vi "Configure Trigger (State).vi"(0 "VISA resource name":refnum<visa-resource-name>, 1 "Trigger Condition (0:False)":u16(ring) items=["False", "True"], 2 "Trigger Event (0:A Event)":u16(ring) items=["A Event", "B Event"], 5 "Channel1 Input":T4={"Channel1 Logical Input (0:High)"=0, "Channel1 Threshold (1.0v)"=1.0} {"Channel1 Logical Input (0:High)" items=["High", "Low", "X"]}, 7 "Channel2 Input":T3={"Channel2 Logical Input (0:High) "=0, "Channel2 Threshold (1.0v) "=1.0} {"Channel2 Logical Input (0:High)" items=["High", "Low", "X"]}, 9 "Pattern Type (0:AND)":u16(ring) items=["AND", "NAND", "OR", "NOR"], 11 "error in (no error)":errorcluster, 12 "Channel3 Input":T2={"Channel3 Logical Input (0:High)"=0, "Channel3 Threshold (1.0v)"=1.0} {"Channel3 Logical Input (0:High)" items=["High", "Low", "X"]}, 13 "Channel4 Input":T1={"Channel4 Logical Input (0:Positive)"=0, "Channel4 Threshold (1.0v)"=1.0} {"Channel4 Logical Input (0:Positive)" items=["Positive", "Negative"]}) -> (4 "VISA resource name out":refnum<visa-resource-name>, 15 "error out":errorcluster)   [LabVIEW 2012, in "Tektronix 7000 Series.lvlib"]
doc: "Configures state trigger settings for an oscilloscope. For a 4-channel oscilloscope, a state occurs when the specified conditions of Channels 1, 2, and 3 are met after the Channel 4 clock condition is met. For a 2-channel oscilloscope, a state occurs when the specified conditions of channel 1 are met after the Channel 2 clock condition is met.\n\nTDS5000,TDS5000B,TDS6000,CSA7000 and TDS7000 series oscilloscopes don't support B State Trigger."
uses:
  Tektronix 7000 Series.lvlib
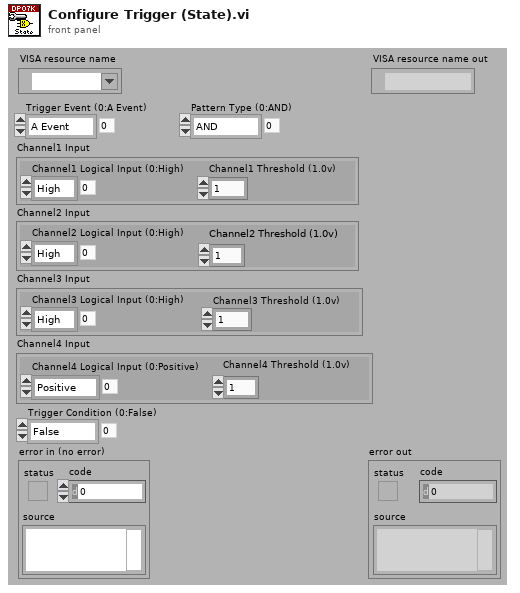
[diagram p1: front panel]
types:
  T1 = cluster{"Channel4 Logical Input (0:Positive)":u16, "Channel4 Threshold (1.0v)":dbl}
  T2 = cluster{"Channel3 Logical Input (0:High)":u16, "Channel3 Threshold (1.0v)":dbl}
  T3 = cluster{"Channel2 Logical Input (0:High) ":u16, "Channel2 Threshold (1.0v) ":dbl}
  T4 = cluster{"Channel1 Logical Input (0:High)":u16, "Channel1 Threshold (1.0v)":dbl}
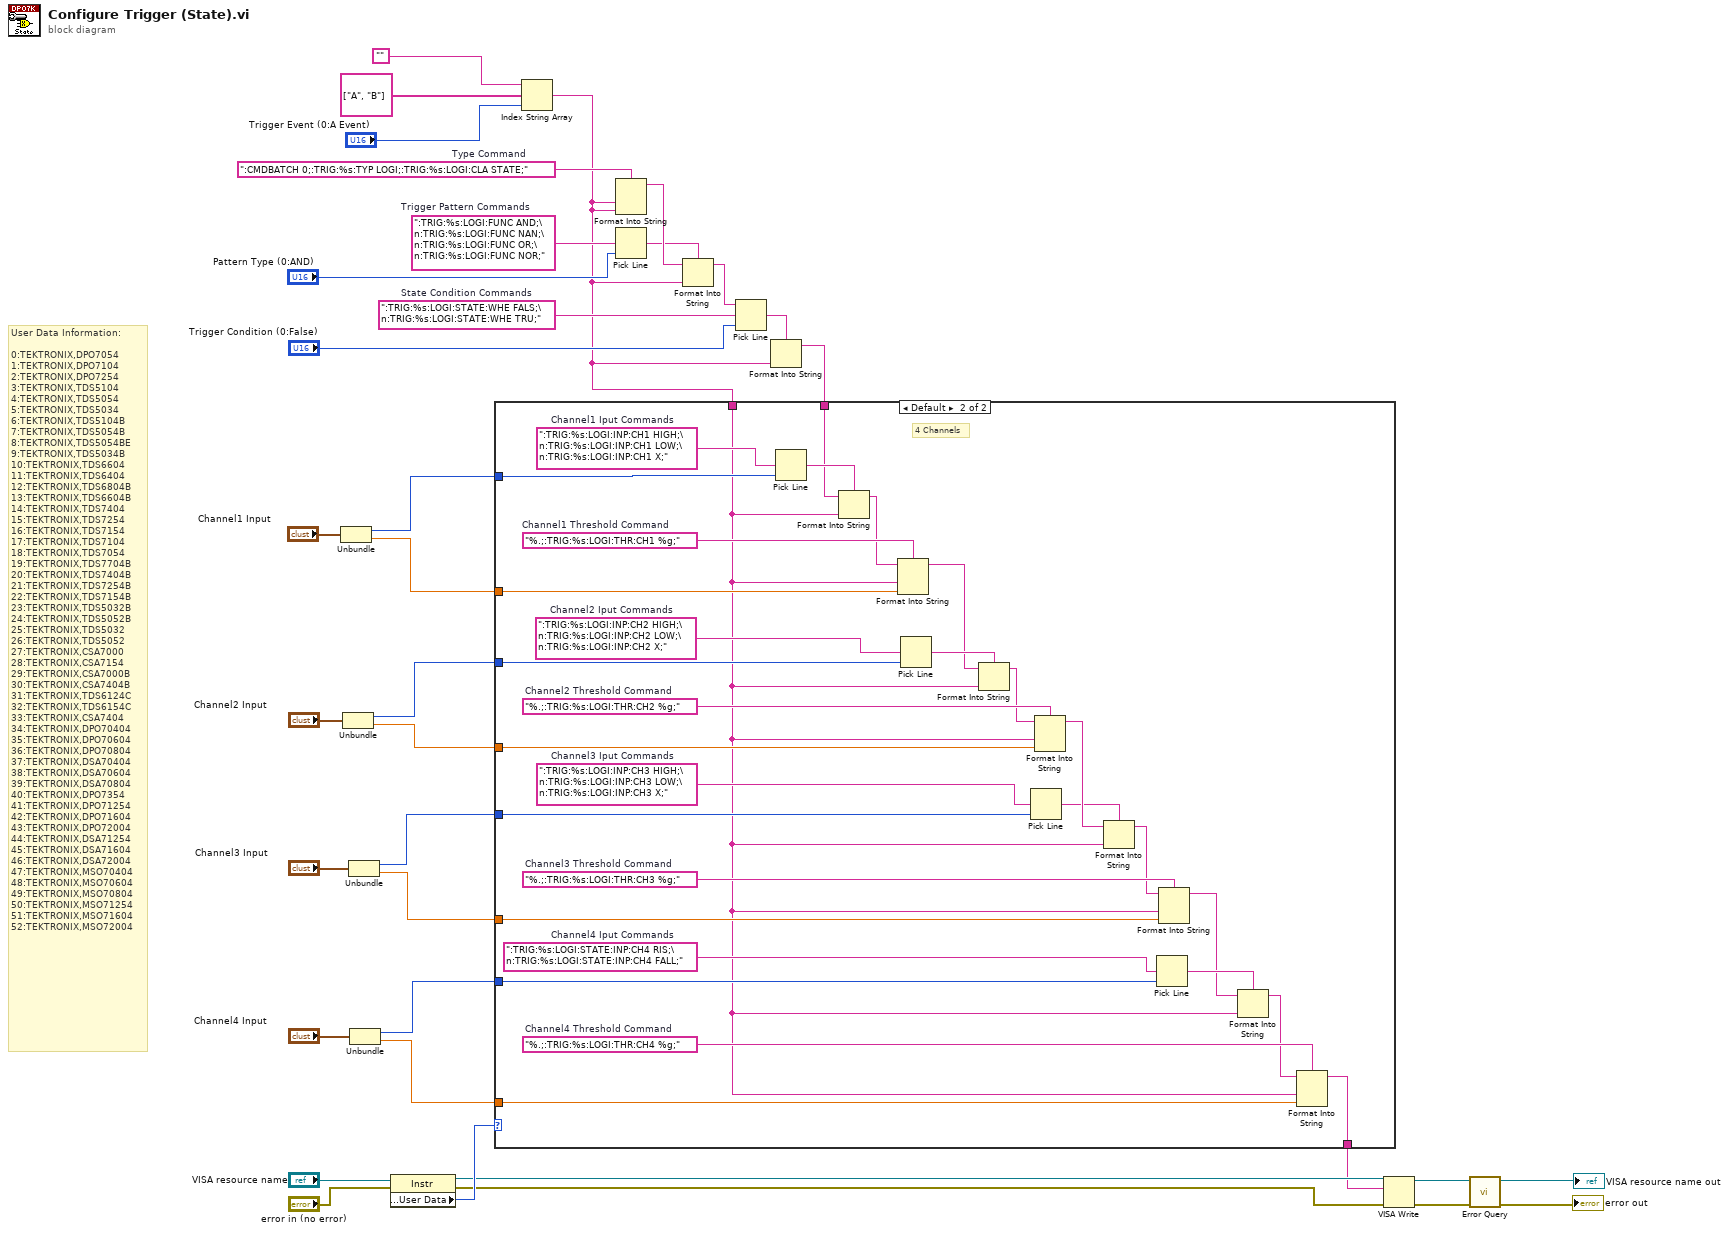
[diagram p0: block diagram]
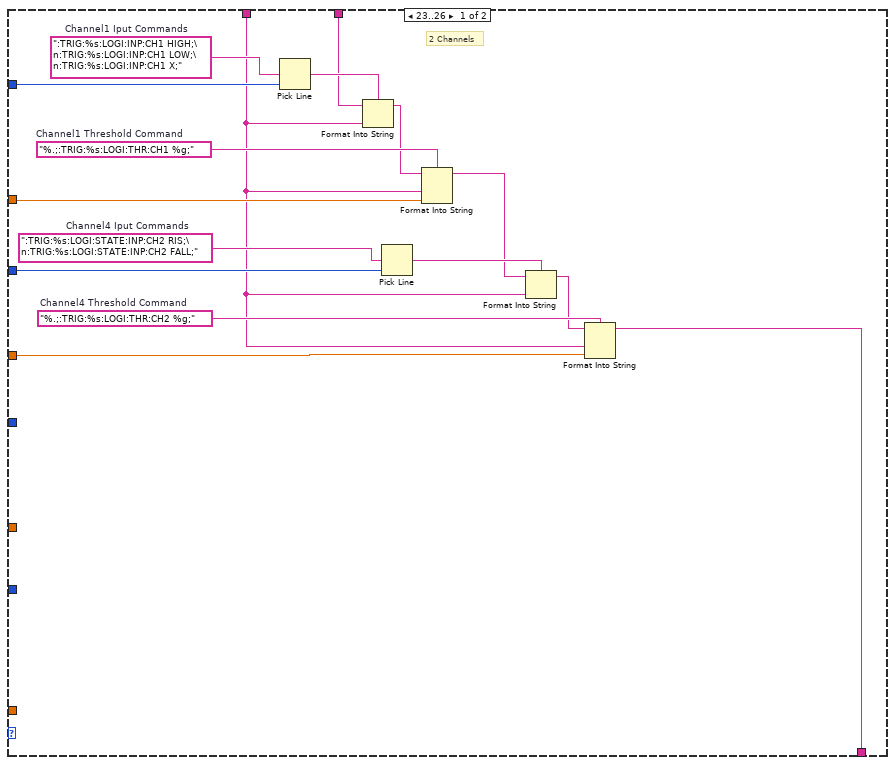
[diagram p2: hidden frame]
diagram:
  w18 = ":TRIG:%s:LOGI:STATE:WHE FALS;\n:TRIG:%s:LOGI:STATE:WHE TRU;"  # State Condition Commands
  w19 = ":TRIG:%s:LOGI:FUNC AND;\n:TRIG:%s:LOGI:FUNC NAN;\n:TRIG:%s:LOGI:FUNC OR;\n:TRIG:%s:LOGI:FUNC NOR;"  # Trigger Pattern Commands
  w17 = ":CMDBATCH 0;:TRIG:%s:TYP LOGI;:TRIG:%s:LOGI:CLA STATE;"  # Type Command
  # "User Data Information:\n\n0:TEKTRONIX,DPO7054\n1:TEKTRONIX,DPO7104\n2:TEKTRONIX,DPO7254\n3:TEKTRONIX,TDS5104\n4:TEKTRONIX,TDS5054\n5:TEKTRONIX,TDS5034\n6:TEKTRONIX,TDS5104B\n7:TEKTRONIX,TDS5054B\n8:TEKTRONIX,TDS5054BE\n9:TEKTRONIX,TDS5034B\n10:TEKTRONIX,TDS6604\n11:TEKTRONIX,TDS6404\n12:TEKTRONIX,TDS6804B\n13:TEKTRONIX,TDS6604B\n14:TEKTRONIX,TDS7404\n15:TEKTRONIX,TDS7254\n16:TEKTRONIX,TDS7154\n17:TEKTRONIX,TDS7104\n18:TEKTRONIX,TDS7054\n19:TEKTRONIX,TDS7704B\n20:TEKTRONIX,TDS7404B\n21:TEKTRONIX,TDS7254B\n22:TEKTRONIX,TDS7154B\n23:TEKTRONIX,TDS5032B\n24:TEKTRONIX,TDS5052B\n25:TEKTRONIX,TDS5032\n26:TEKTRONIX,TDS5052\n27:TEKTRONIX,CSA7000\n28:TEKTRONIX,CSA7154\n29:TEKTRONIX,CSA7000B\n30:TEKTRONIX,CSA7404B\n31:TEKTRONIX,TDS6124C\n32:TEKTRONIX,TDS6154C\n33:TEKTRONIX,CSA7404\n34:TEKTRONIX,DPO70404\n35:TEKTRONIX,DPO70604\n36:TEKTRONIX,DPO70804\n37:TEKTRONIX,DSA70404\n38:TEKTRONIX,DSA70604\n39:TEKTRONIX,DSA70804\n40:TEKTRONIX,DPO7354\n41:TEKTRONIX,DPO71254\n42:TEKTRONIX,DPO71604\n43:TEKTRONIX,DPO72004\n44:TEKTRONIX,DSA71254\n45:TEKTRONIX,DSA71604\n46:TEKTRONIX,DSA72004\n47:TEKTRONIX,MSO70404\n48:TEKTRONIX,MSO70604\n49:TEKTRONIX,MSO70804\n50:TEKTRONIX,MSO71254\n51:TEKTRONIX,MSO71604\n52:TEKTRONIX,MSO72004"
  n1 = Unbundle("Channel1 Input") -> ("Channel1 Logical Input (0:High)"=w34:u16, "Channel1 Threshold (1.0v)"=w14:dbl)
  n2 = Unbundle("Channel2 Input") -> ("Channel2 Logical Input (0:High)"=w32:u16, "Channel2 Threshold (1.0v)"=w13:dbl)
  n3 = Unbundle("Channel3 Input") -> ("Channel3 Logical Input (0:High)"=w30:u16, "Channel3 Threshold (1.0v)"=w12:dbl)
  n4 = Unbundle("Channel4 Input") -> ("Channel4 Logical Input (0:Positive)"=w28:u16, "Channel4 Threshold (1.0v)"=w11:dbl)
  n5 = property class="Instr"(reference="VISA resource name", error in="error in (no error)") -> (reference out=w4:refnum<visa-resource-name>, error out=w3:errorcluster, "General Settings:User Data"=w5:u32)
  n6 = Index String Array(1:"Trigger Event (0:A Event)", 2:string[] ["A", "B"], 3:"" ("Empty String Constant")) -> (0:w8:string)
  n7 = Format Into String(format string=w17, w8, w8) -> (resulting string=w16:string)  [unwired: 2 in, 1 out]
  n8 = Pick Line(multi-line string=w19, line index="Pattern Type (0:AND)") -> (output string=w15:string)  [unwired: 1 in]
  n9 = Format Into String(format string=w15, initial string=w16, w8) -> (resulting string=w9:string)  [unwired: 1 in, 1 out]
  n10 = Pick Line(string ("")=w9, multi-line string=w18, line index="Trigger Condition (0:False)") -> (output string=w10:string)
  n11 = Format Into String(format string=w10, w8) -> (resulting string=w1:string)  [unwired: 2 in, 1 out]
  n12 = case shown="Default" w5 {
    tunnel: w34 -> [w48 w82]
    tunnel: w32 -> [w41 w81]
    tunnel: w30 -> [_ w80]
    tunnel: w28 -> [_ w79]
    tunnel: w14 -> [w47 w68]
    tunnel: w13 -> [w42 w64]
    tunnel: w12 -> [_ w60]
    tunnel: w11 -> [_ w56]
    tunnel: w8 -> [w40 w55]
    tunnel: [w38 w54] -> w2
    tunnel: w1 -> [w37 w53]
    frame 23..26 {
      w46 = "%.;:TRIG:%s:LOGI:THR:CH2 %g;"  # Channel4 Threshold Command
      w45 = ":TRIG:%s:LOGI:STATE:INP:CH2 RIS;\n:TRIG:%s:LOGI:STATE:INP:CH2 FALL;"  # Channel4 Iput Commands
      w51 = "%.;:TRIG:%s:LOGI:THR:CH1 %g;"  # Channel1 Threshold Command
      w52 = ":TRIG:%s:LOGI:INP:CH1 HIGH;\n:TRIG:%s:LOGI:INP:CH1 LOW;\n:TRIG:%s:LOGI:INP:CH1 X;"  # Channel1 Iput Commands
      # "2 Channels"
      n13 = Pick Line(multi-line string=w52, line index=w48) -> (output string=w50:string)  [unwired: 1 in]
      n14 = Format Into String(format string=w50, initial string=w37, w40) -> (resulting string=w49:string)  [unwired: 1 in, 1 out]
      n15 = Pick Line(multi-line string=w45, line index=w41) -> (output string=w44:string)  [unwired: 1 in]
      n16 = Format Into String(format string=w51, initial string=w49, w40, w47) -> (resulting string=w39:string)  [unwired: 1 in, 1 out]
      n17 = Format Into String(format string=w44, initial string=w39, w40) -> (resulting string=w43:string)  [unwired: 1 in, 1 out]
      n18 = Format Into String(format string=w46, initial string=w43, w40, w42) -> (resulting string=w38:string)  [unwired: 1 in, 1 out]
    }
    frame Default {
      w72 = "%.;:TRIG:%s:LOGI:THR:CH4 %g;"  # Channel4 Threshold Command
      w71 = ":TRIG:%s:LOGI:STATE:INP:CH4 RIS;\n:TRIG:%s:LOGI:STATE:INP:CH4 FALL;"  # Channel4 Iput Commands
      w73 = "%.;:TRIG:%s:LOGI:THR:CH3 %g;"  # Channel3 Threshold Command
      w74 = ":TRIG:%s:LOGI:INP:CH3 HIGH;\n:TRIG:%s:LOGI:INP:CH3 LOW;\n:TRIG:%s:LOGI:INP:CH3 X;"  # Channel3 Iput Commands
      w76 = "%.;:TRIG:%s:LOGI:THR:CH2 %g;"  # Channel2 Threshold Command
      w75 = ":TRIG:%s:LOGI:INP:CH2 HIGH;\n:TRIG:%s:LOGI:INP:CH2 LOW;\n:TRIG:%s:LOGI:INP:CH2 X;"  # Channel2 Iput Commands
      w77 = "%.;:TRIG:%s:LOGI:THR:CH1 %g;"  # Channel1 Threshold Command
      w78 = ":TRIG:%s:LOGI:INP:CH1 HIGH;\n:TRIG:%s:LOGI:INP:CH1 LOW;\n:TRIG:%s:LOGI:INP:CH1 X;"  # Channel1 Iput Commands
      # "4 Channels"
      n19 = Pick Line(multi-line string=w78, line index=w82) -> (output string=w70:string)  [unwired: 1 in]
      n20 = Format Into String(format string=w70, initial string=w53, w55) -> (resulting string=w69:string)  [unwired: 1 in, 1 out]
      n21 = Format Into String(format string=w77, initial string=w69, w55, w68) -> (resulting string=w66:string)  [unwired: 1 in, 1 out]
      n22 = Pick Line(multi-line string=w75, line index=w81) -> (output string=w67:string)  [unwired: 1 in]
      n23 = Format Into String(format string=w67, initial string=w66, w55) -> (resulting string=w65:string)  [unwired: 1 in, 1 out]
      n24 = Pick Line(multi-line string=w74, line index=w80) -> (output string=w62:string)  [unwired: 1 in]
      n25 = Format Into String(format string=w76, initial string=w65, w55, w64) -> (resulting string=w63:string)  [unwired: 1 in, 1 out]
      n26 = Format Into String(format string=w62, initial string=w63, w55) -> (resulting string=w61:string)  [unwired: 1 in, 1 out]
      n27 = Pick Line(multi-line string=w71, line index=w79) -> (output string=w59:string)  [unwired: 1 in]
      n28 = Format Into String(format string=w73, initial string=w61, w55, w60) -> (resulting string=w58:string)  [unwired: 1 in, 1 out]
      n29 = Format Into String(format string=w59, initial string=w58, w55) -> (resulting string=w57:string)  [unwired: 1 in, 1 out]
      n30 = Format Into String(format string=w72, initial string=w57, w55, w56) -> (resulting string=w54:string)  [unwired: 1 in, 1 out]
    }
  }
  n31 = VISA Write(VISA resource name=w4, write buffer=w2, error in (no error)=w3) -> (VISA resource name out=w25:refnum<visa-resource-name>, error out=w26:errorcluster)  [unwired: 1 out]
  n32 = call "Error Query.vi"("error in (no error)"=w26, "VISA resource name"=w25) -> ("error out"=→"error out":errorcluster, "VISA resource name out"=→"VISA resource name out":refnum<visa-resource-name>)  [unwired: 6 in, 2 out]
